vi "shape1.vi"() -> ()   [LabVIEW 2020]
uses:
  bee2abb7-c490-4ad6-bfc0-30ed72578e14.vi
panel:
  out "Array":cluster{"x":dbl, "y":dbl}[](array[cluster])
  in  "input variable":dbl=5.5 format="%#_13g"
  out "XY Graph":cluster{dbl[], dbl[]}(graph)
  # "e"
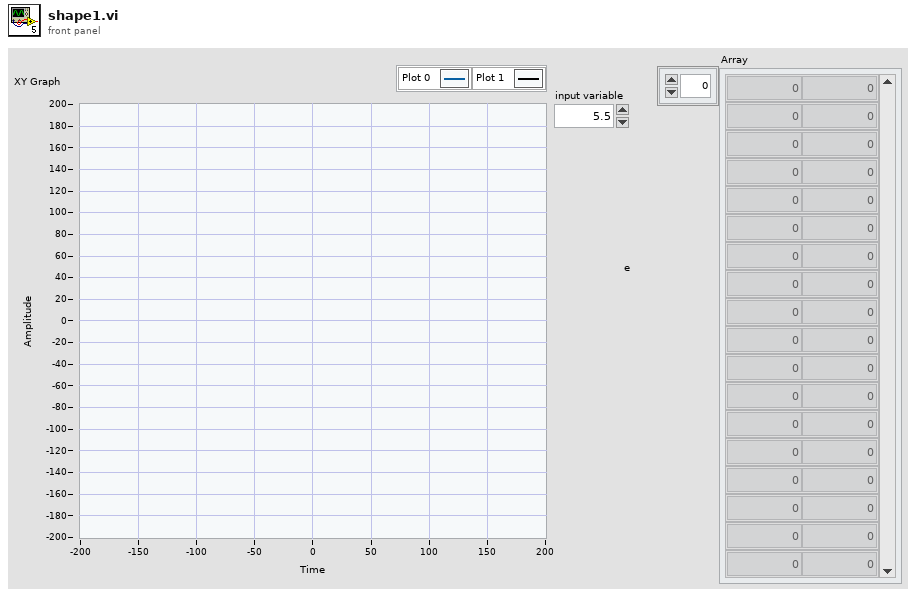
[diagram p1: front panel]
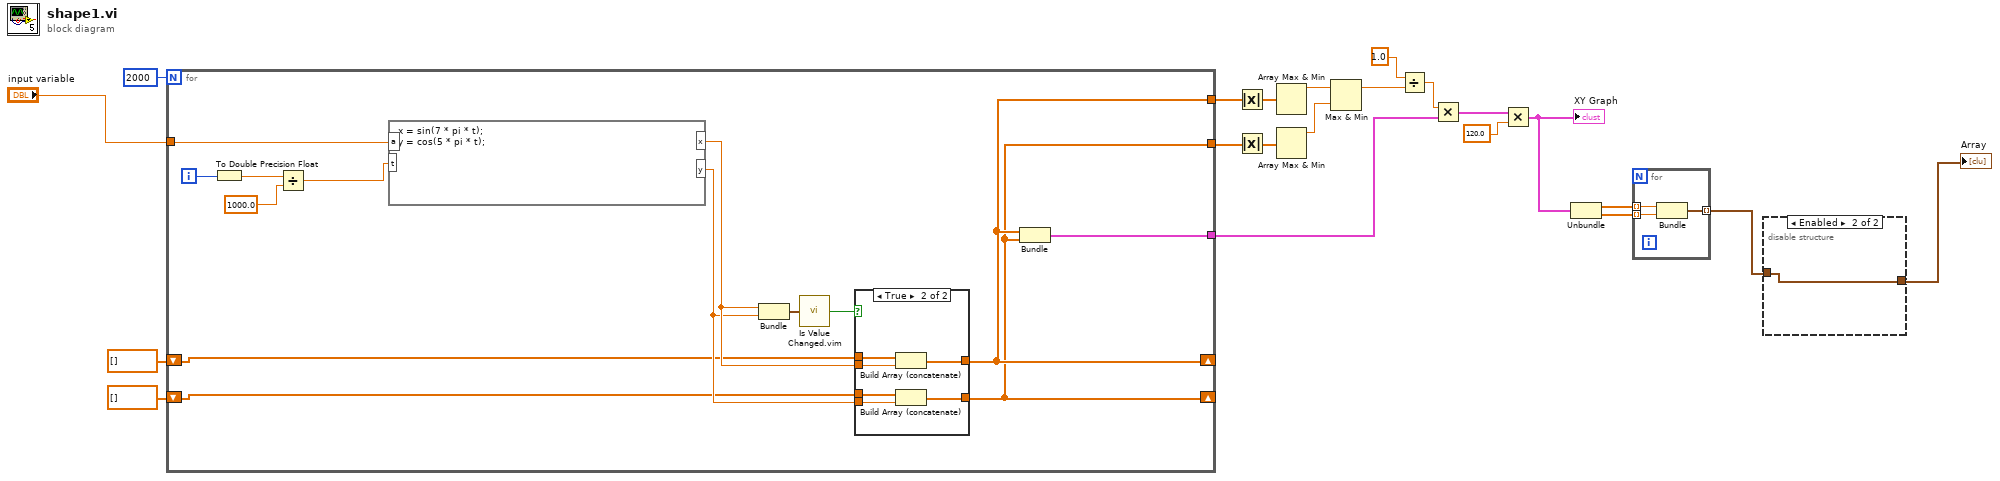
[diagram p0: block diagram]
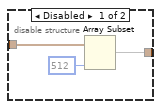
[diagram p2: hidden frame]
diagram:
  n1 = for {
    N: 2000 -> [_]
    tunnel: "input variable" -> [w35]
    shift-right: [w23] -> _
    shift-left: dbl[] [] -> [w30]
    shift-right: [w22] -> _
    shift-left: dbl[] [] -> [w29]
    tunnel: [w28] -> w8
    tunnel: [w23] -> w17
    tunnel: [w22] -> w16
    i -> [w27]
    n2 = To Double Precision Float(number=w27) -> (double precision float=w26:dbl)
    n3 = Divide(x=w26, y=1000.0) -> (x/y=w24:dbl)
    n4 = formula code="x = sin(7 * pi * t);\ny = cos(5 * pi * t);"("a"=w35, "t"=w24) -> ("x"=w32:dbl, "y"=w31:dbl)
    n5 = Bundle("x"=w32, "y"=w31) -> (w34:cluster{"x":dbl, "y":dbl})  [unwired: 1 in]
    n6 = call "Is Value Changed.vim"("value"=w34) -> ("changed or first call?"=w33:bool)
    n7 = case shown="True" w33 {
      tunnel: w32 -> [_ w43]
      tunnel: w31 -> [_ w42]
      tunnel: [w37 w41] -> w23
      tunnel: [w36 w40] -> w22
      tunnel: w30 -> [w37 w39]
      tunnel: w29 -> [w36 w38]
      frame False {
      }
      frame True {
        n8 = Build Array (concatenate)(w39, w43) -> (w41:dbl[])
        n9 = Build Array (concatenate)(w38, w42) -> (w40:dbl[])
      }
    }
    n10 = Bundle(w23, w22) -> (w28:cluster{dbl[], dbl[]})  [unwired: 1 in]
  }
  n11 = Absolute Value(x=w17) -> (abs(x)=w15:dbl[])
  n12 = Absolute Value(x=w16) -> (abs(x)=w14:dbl[])
  n13 = Array Max & Min(array=w15) -> (max value=w13:dbl)  [unwired: 3 out]
  n14 = Array Max & Min(array=w14) -> (max value=w12:dbl)  [unwired: 3 out]
  n15 = Max & Min(x=w13, y=w12) -> (max(x,y)=w11:dbl)  [unwired: 1 out]
  n16 = Divide(x=1.0, y=w11) -> (x/y=w9:dbl)
  n17 = Multiply(x=w9, y=w8) -> (x*y=w7:cluster{dbl[], dbl[]})
  n18 = Multiply(x=w7, y=120.0 ("x")) -> (x*y=w5:cluster{dbl[], dbl[]})
  "XY Graph" <- w5
  n19 = Unbundle(w5) -> (w4:dbl[], w3:dbl[])
  n20 = for {
    tunnel: w4 -> [w46] mode=indexing
    tunnel: w3 -> [w45] mode=indexing
    tunnel: [w44] -> w2 mode=indexing
    n21 = Bundle("x"=w46, "y"=w45) -> (w44:cluster{"x":dbl, "y":dbl})  [unwired: 1 in]
  }
  n22 = disable-structure shown="Enabled" {
    disable-tunnel: w2 -> [w49 w50]
    disable-tunnel: [w47 w50] -> w1
    frame Disabled {
      n23 = Array Subset(array=w49, length=512) -> (w47:cluster{"x":dbl, "y":dbl}[])  [unwired: 1 in]
    }
    frame Enabled {
    }
  }
  "Array" <- w1
